vi "查找可用串口.vi"(1 "配置检索参数":T1={"发送指令"="+TXYBJT TECH", "等待时间（毫秒）"=500, "响应数据"="DTU Software,VER", "波特率"=[1200, 2400, 4800, 9600, 19200]}) -> (0 "已检索串口参数":T3={"COM号"="", "波特率"=9600, "数据比特"=8, "奇偶"=enum."None", "停止位"=10, "流控制"=0} {"流控制" items=["无"=0, "XON/XOFF"=1, "RTS/CTS"=2, "DTR/DSR"=4]; "停止位" items=["1.0"=10, "1.5"=15, "2.0"=20]; "波特率" items=["75"=75, "110"=110, "134"=134, "150"=150, "300"=300, "600"=600, "1200"=1200, "1800"=1800, "2400"=2400, "4800"=4800, "7200"=7200, "9600"=9600, "14400"=14400, "19200"=19200, "28800"=28800, "38400"=38400, "56000"=56000, "57600"=57600, "115200"=115200, "128000"=128000, "230400"=230400]})   [LabVIEW 2015]
uses:
  Serial - Settings.ctl
  <vilib>/Instr/_visa.llb/VISA Find Search Mode.ctl
panel:
  out "检索进程":i32(slide) max=6 scale=0.0..6.0
  out "调用时间":dbl
  # "使用模块：\nDW02xx系列GPRS模块\n\n使用方法：\n自动进行检索模块\n\n用户须知：\n1、确保模块连接串口\n2、确保模块供电，EN置高\n3、完成后自动退出"
  # "<10s"
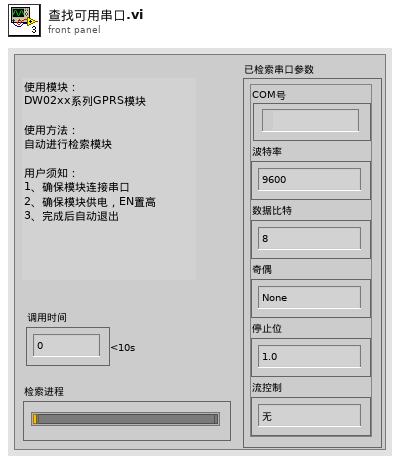
[diagram p1: front panel]
types:
  T1 = typedef "检索模块.ctl" = cluster{"发送指令":string, "等待时间（毫秒）":u32, "响应数据":string, "波特率":T2}
  T2 = typedef "波特率.ctl" = u32[]
  T3 = typedef "Serial - Settings.ctl" = cluster{"COM号":refnum<visa-resource-name>, "波特率":u32, "数据比特":u16, "奇偶":enum16{"None", "Odd", "Even", "Mark", "Space"}, "停止位":u16, "流控制":u16}
  T4 = typedef "VISA Find Search Mode.ctl" = u32
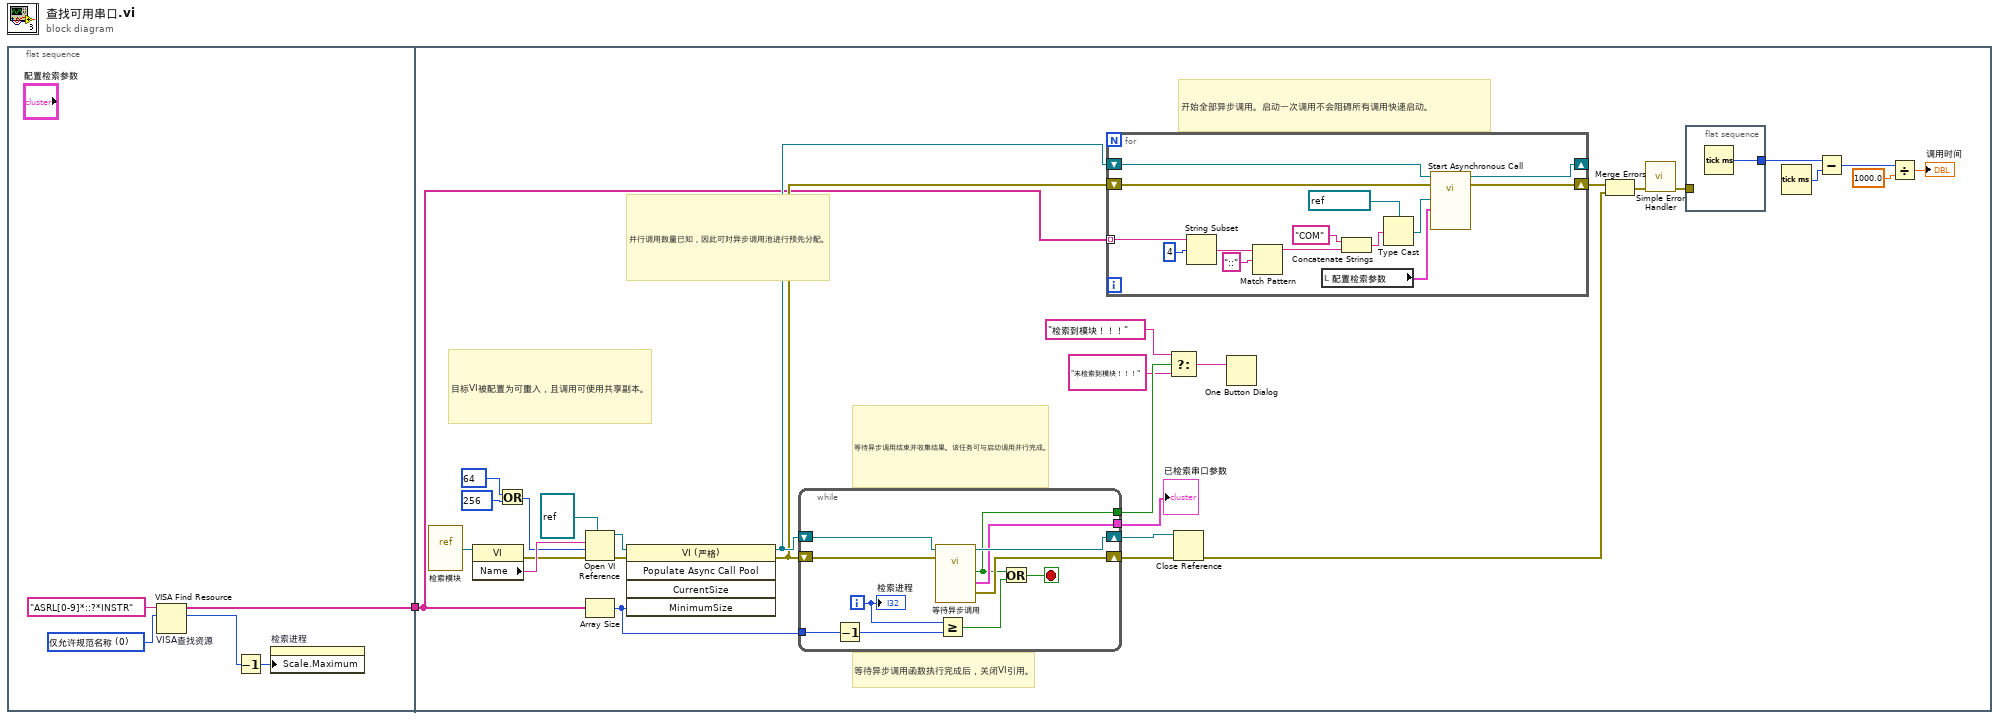
[diagram p0: block diagram]
diagram:
  n1 = flat-sequence {
    tunnel: [w2] -> w1
    tunnel: w1 -> [w8]
    frame #0 {
      w3 = T4 0 items=["仅允许规范名称"=0, "只允许别名"=2, "包含匹配别名"=3, "包含所有别名"=4] ("Search Mode")
      n2 = VISA Find Resource "VISA查找资源"(10:w3, 11:"ASRL[0-9]*::?*INSTR" ("表达式(\"?*\")")) -> (2:w6:u32, 3:w2:string[])  [unwired: 1 in, 1 out]
      n3 = Decrement(x=w6) -> (x-1=w5:u32)
      n4 = property on="检索进程" class="Slide (严格)"("Scale.Maximum"=w5) -> ()  [unwired: 2 in, 2 out]
    }
    frame #1 {
      # "等待异步调用函数执行完成后，关闭VI引用。"
      # "开始全部异步调用。启动一次调用不会阻碍所有调用快速启动。"
      # "等待异步调用结束并收集结果。该任务可与启动调用并行完成。"
      # "并行调用数量已知，因此可对异步调用池进行预先分配。"
      # "目标VI被配置为可重入，且调用可使用共享副本。"
      n5 = vi-ref "检索模块.vi"() -> (w17:refnum<vi>)
      n6 = property class="VI"(reference=w17) -> (error out=w16:errorcluster, "Name"=w35:string)  [unwired: 1 in, 1 out]
      n7 = Or(x=64 ("options"), y=256 ("options")) -> (x .or. y?=w18:i32)
      n8 = Open VI Reference(type specifier VI Refnum (for type only)=refnum<vi> refnum, vi path=w35, options=w18, error in (no error)=w16) -> (vi reference=w27:refnum<vi>, error out=w26:errorcluster)  [unwired: 2 in]
      n9 = Array Size(array=w8) -> (size(s)=w15:i32)
      n10 = invoke class="VI (严格)" method="Populate Async Call Pool"(reference=w27, error in=w26, "MinimumSize"=w15) -> (reference out=w25:refnum<vi>, error out=w24:errorcluster)  [unwired: 2 in, 3 out]
      n11 = while {
        shift-right: [w44] -> w28
        shift-left: w25 -> [w46]
        shift-right: [w43] -> w21
        shift-left: w24 -> [w45]
        tunnel: w15 -> [w40]
        tunnel: [w37] -> w14
        tunnel: [w36] -> w13
        i -> [w38]
        stop <- w41 stop-if-true
        n12 = Decrement(x=w40) -> (x-1=w39:i32)
        n13 = call-by-ref "等待异步调用"(reference=w46, error in=w45) -> (reference out=w44:refnum<vi>, "错误输出"=w43:errorcluster, "串口参数输出"=w37:T3, "isfind？"=w36:bool)  [unwired: 3 in, 1 out]
        n14 = Greater Or Equal?(x=w38, y=w39) -> (x >= y?=w42:bool)
        n15 = Or(x=w36, y=w42) -> (x .or. y?=w41:bool)
        "检索进程" <- w38
      }
      "已检索串口参数" <- w14
      n16 = for {
        tunnel: w8 -> [w55] mode=indexing
        shift-right: [w59] -> w23
        shift-left: w24 -> [w60]
        shift-right: [w57] -> _
        shift-left: w25 -> [w58]
        n17 = String Subset(string=w55, offset (0)=4 ("偏移量(0)")) -> (substring=w53:string)  [unwired: 1 in]
        n18 = Match Pattern(string=w53, regular expression="::" ("正则表达式")) -> (before substring=w51:string)  [unwired: 1 in, 3 out]
        n19 = local read "配置检索参数"() -> (w48:T1)
        n20 = Concatenate Strings("COM" ("字符串"), w51) -> (w49:string)
        n21 = Type Cast(type=refnum<visa-resource-name> "COM1" ("COM号"), x=w49) -> (*(type *) &x=w47:refnum<visa-resource-name>)
        n22 = call-by-ref "Start Asynchronous Call"(reference=w58, error in=w60, "检索参数配置输入"=w48, "COM号"=w47) -> (reference out=w57:refnum<vi>, error out=w59:errorcluster)  [unwired: 1 in, 3 out]
      }
      n23 = Select(t="检索到模块！！！", s=w13, f="未检索到模块！！！") -> (s? t:f=w12:string)
      n24 = Close Reference(reference=w28, error in (no error)=w21) -> (error out=w22:errorcluster)
      n25 = One Button Dialog(message=w12) -> ()  [unwired: 1 in, 1 out]
      n26 = Merge Errors(w23, w22) -> (w34:errorcluster)
      n27 = call <vilib>:"Simple Error Handler.vi"("error in (no error)"=w34) -> ("error out"=w9:errorcluster)  [unwired: 4 in, 4 out]
      n28 = flat-sequence {
        tunnel: [w61] -> w31
        tunnel: w9 -> [_]
        frame #0 {
          n29 = Tick Count (ms)() -> (millisecond timer value=w61:u32)
        }
      }
      n30 = Tick Count (ms)() -> (millisecond timer value=w30:u32)
      n31 = Subtract(x=w31, y=w30) -> (x-y=w33:u32)
      n32 = Divide(x=w33, y=1000.0) -> (x/y=→"调用时间":dbl)
    }
  }
